vi "Update Series Graphs.vi"(8 "error in (no error)":errorcluster, 9 "Image #":u32, 10 "Image Series":u16[][][](array[numeric]), 11 "Series Graph in":refnum<class "Series Graph.lvclass">) -> (0 "error out":errorcluster, 3 "Series Graph out":refnum<class "Series Graph.lvclass">)   [LabVIEW 2023, in "Series Graph.lvclass"]
uses:
  Series Graph.lvclass
  Series Graph.lvclass/Series Graph.ctl
  Detail Graph/Detail Graph.lvclass
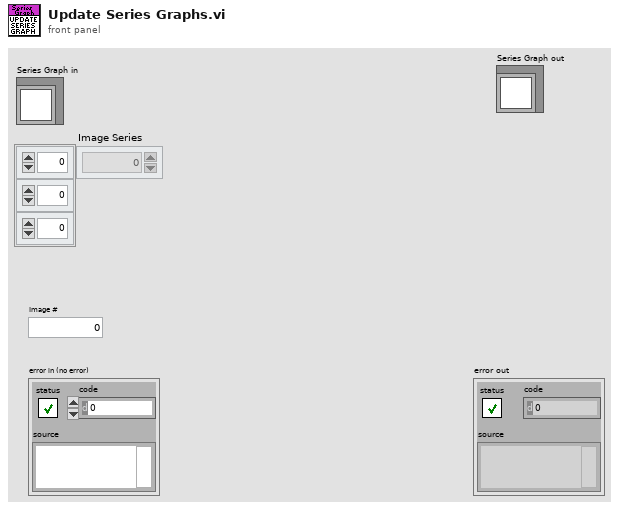
[diagram p1: front panel]
types:
  T1 = typedef "LVPointDoubleTypeDef.ctl" = cluster{"X":dbl, "Y":dbl}
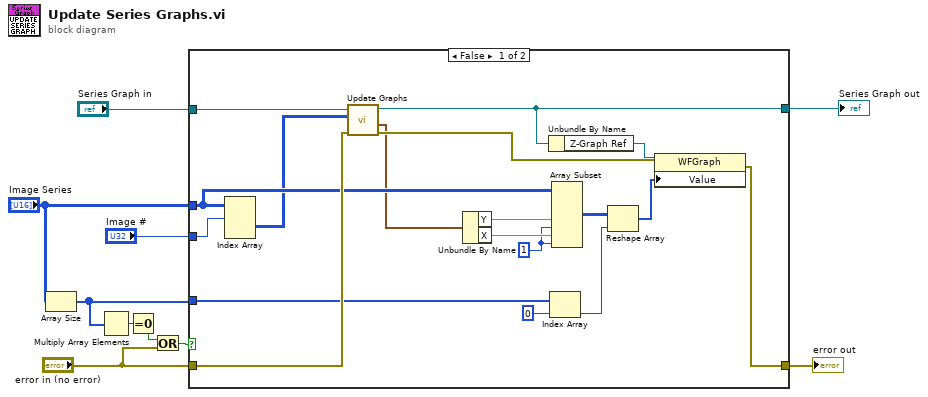
[diagram p0: block diagram]
diagram:
  n1 = Array Size(array="Image Series") -> (size(s)=w3:i32[])
  n2 = Multiply Array Elements(1:w3) -> (0:w8:i32)
  n3 = Equal To 0?(x=w8) -> (x = 0?=w6:bool)
  n4 = Or(x=w6, y="error in (no error)") -> (x .or. y?=w7:bool)
  n5 = case shown="False" w7 {
    tunnel: [w15 w30] -> w10
    tunnel: [w13 w29] -> w1
    tunnel: "Image Series" -> [w24 _]
    tunnel: "Image #" -> [w28 _]
    tunnel: "error in (no error)" -> [w27 w30]
    tunnel: w3 -> [w26 _]
    tunnel: "Series Graph in" -> [w14 w29]
    frame False {
      w21 = 1 ("length")
      n6 = Index Array(array=w24, index (dim 0)=w28) -> (element=w12:u16[][])  [unwired: 2 in]
      n7 = call "Update Graphs.vi"("error in (no error)"=w27, "image"=w12, "Detail Graph in"=w14) -> ("error out"=w16:errorcluster, "Cursor.Cursor Position"=w11:T1, "Detail Graph out"=w13:refnum<class "Series Graph.lvclass">)  [unwired: 6 in]
      n8 = Unbundle By Name(w11) -> ("Y"=w23:dbl, "X"=w22:dbl)
      n9 = Unbundle By Name(w13) -> ("Z-Graph Ref"=w18:refnum<vi>)
      n10 = Index Array(array=w26, index=0) -> (element=w19:i32)
      n11 = Array Subset(array=w24, index (dim 1)=w23, length (dim 1)=w21, index (dim 2)=w22, length (dim 2)=w21) -> (w20:u16[][][])  [unwired: 2 in]
      n12 = Reshape Array(w20, w19) -> (w17:u16[])
      n13 = property class="WFGraph"(reference=w18, error in=w16, "Value"=w17) -> (error out=w15:errorcluster)  [unwired: 1 out]
    }
    frame True {
    }
  }
  "error out" <- w10
  "Series Graph out" <- w1
